vi "Configure External Mixer.vi"(0 "VISA resource name":refnum<visa-resource-name>, 5 "Enable External Mixer (F:Disable)":bool, 7 "External Mixer Band (0:Free Run)":i32(ring) items=["A+", "Q+", "U+", "V+", "E+", "W+", "F+", "D+", "G+", "Y+", "J+"], 9 "Mixer Bias (0.0mA)":dbl min=0.0 max=20.0, 11 "error in (no error)":errorcluster, 12 "Conversion Loss (15.0dB)":dbl=15.0 min=0.0 max=99.99) -> (4 "VISA resource name out":refnum<visa-resource-name>, 15 "error out":errorcluster)   [LabVIEW 2020, in "Anritsu Signal Analyzer Series.lvlib"]
doc: "Configures the external mixer settings of the spectrum analyzer."
uses:
  Anritsu Signal Analyzer Series.lvlib
panel:
  # "mA"
  # "dB"
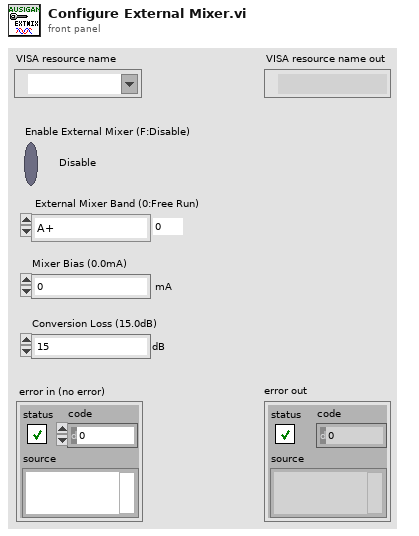
[diagram p1: front panel]
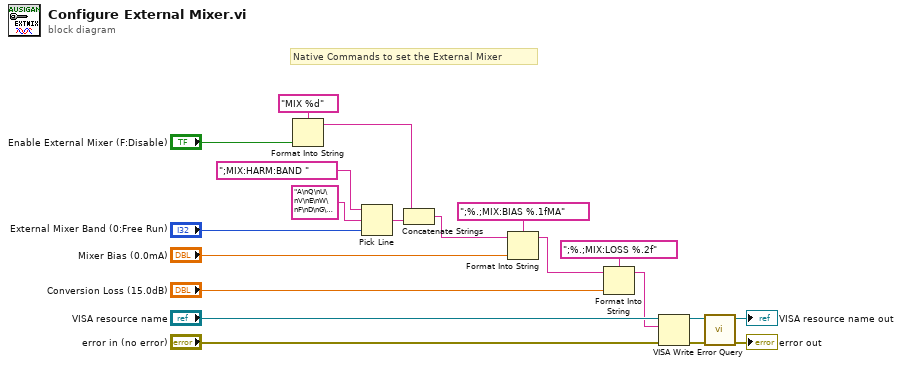
[diagram p0: block diagram]
diagram:
  # "Native Commands to set the External Mixer"
  n1 = Format Into String(format string="MIX %d", "Enable External Mixer (F:Disable)") -> (resulting string=w4:string)  [unwired: 2 in, 1 out]
  n2 = Pick Line(string ("")=";MIX:HARM:BAND ", multi-line string="A\nQ\nU\nV\nE\nW\nF\nD\nG\nY\nJ", line index="External Mixer Band (0:Free Run)") -> (output string=w5:string)
  n3 = Concatenate Strings(w4, w5) -> (w3:string)
  n4 = Format Into String(format string=";%.;MIX:BIAS %.1fMA" ("Format String"), initial string=w3, "Mixer Bias (0.0mA)") -> (resulting string=w2:string)  [unwired: 1 in, 1 out]
  n5 = Format Into String(format string=";%.;MIX:LOSS %.2f" ("Format String"), initial string=w2, "Conversion Loss (15.0dB)") -> (resulting string=w1:string)  [unwired: 1 in, 1 out]
  n6 = VISA Write(VISA resource name="VISA resource name", write buffer=w1, error in (no error)="error in (no error)") -> (VISA resource name out=w15:refnum<visa-resource-name>, error out=w16:errorcluster)  [unwired: 1 out]
  n7 = call "Error Query.vi"("error in (no error)"=w16, "VISA resource name"=w15) -> ("error out"=→"error out":errorcluster, "VISA resource name out"=→"VISA resource name out":refnum<visa-resource-name>)  [unwired: 6 in, 2 out]
